vi "MDF4 Add Channel (Double).vi"(4 "Channel Unit":string, 5 "Channel Name":string, 6 "chan_index":u64, 7 "path in":path, 8 "Error In":errorcluster, 9 "Channel Group Reference in":i64, 10 "Data Group Reference in":i64, 11 "MDF4 File Reference in":i64) -> (0 "Error Out":errorcluster, 2 "Data Group Reference out":i64, 3 "MDF4 File Reference out":i64)   [LabVIEW 2019, in "MD4Logger Engine.lvlib"]
uses:
  MD4Logger Engine.lvlib
  <vilib>/Utility/error.llb/Error Cluster From Error Code.vi
  <vilib>/ErrorRing/Error Ring.xnode
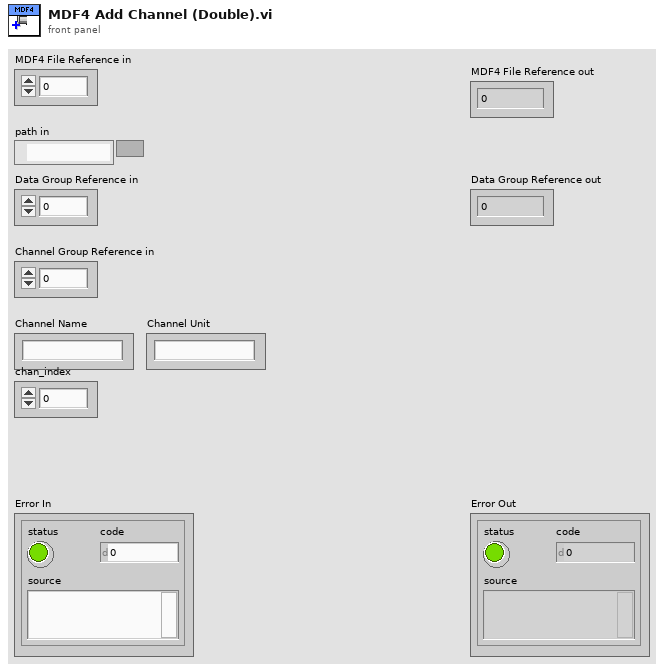
[diagram p1: front panel]
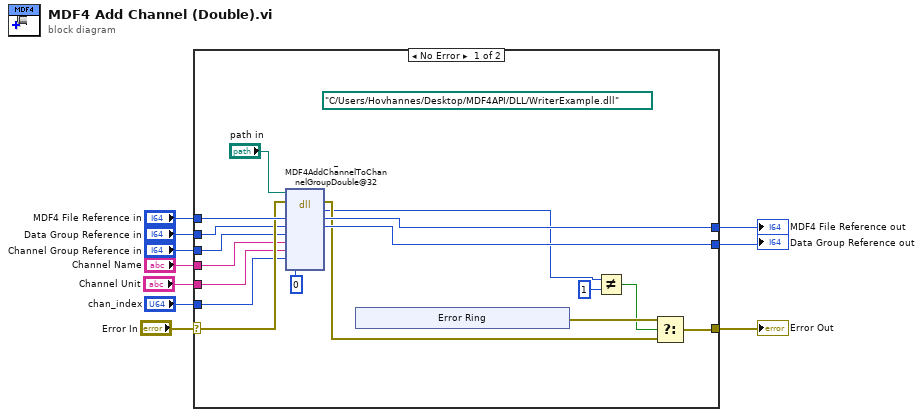
[diagram p0: block diagram]
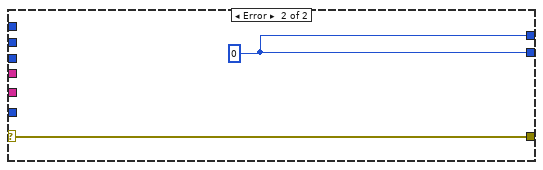
[diagram p2: hidden frame]
diagram:
  n1 = case shown="No Error" "Error In" {
    selector: "Error In" -> [w26 w34]
    tunnel: "MDF4 File Reference in" -> [w27 _]
    tunnel: [w21 w34] -> w8
    tunnel: [w25 w33] -> w7
    tunnel: [w24 w33] -> w6
    tunnel: "Data Group Reference in" -> [w23 _]
    tunnel: "Channel Group Reference in" -> [w19 _]
    tunnel: "Channel Name" -> [w18 _]
    tunnel: "chan_index" -> [w17 _]
    tunnel: "Channel Unit" -> [w11 _]
    frame No Error {
      (unwired) path "C:/Users/Hovhannes/Desktop/MDF4API/DLL/WriterExample.dll" ("path in")
      n2 = dll-call lib="C:/Users/Hovhannes/Desktop/MD4Logger/Source/Engine/DLL/WriterExample.dll" fn="_MDF4AddChannelToChannelGroupDouble@32"(path in="path in", error in=w26, "m4"=w27, "dg"=w23, "cg"=w19, "channel_name"=w18, "channel_unit"=w11, "chan_index"=w17, "cn"=i64 0) -> (error out=w20:errorcluster, "return type"=w15:i32, "m4"=w24:i64, "dg"=w25:i64)  [unwired: 6 in, 1 out]
      n3 = xnode "Error Ring"() -> ("error out"=w22:errorcluster)
      n4 = Not Equal?(x=w15, y=1) -> (x != y?=w14:bool)
      n5 = Select(t=w22, s=w14, f=w20) -> (s? t:f=w21:errorcluster)
    }
    frame Error {
      w33 = i64 0 ("m4")
    }
  }
  "Data Group Reference out" <- w7
  "Error Out" <- w8
  "MDF4 File Reference out" <- w6
